vi "File.Move with Overwrite.vi"(8 "error in (no error)":errorcluster, 10 "Destination":path, 11 "Source":path) -> (0 "error out":errorcluster, 2 "Files Moved":i32, 3 "Destination Dup":path)   [LabVIEW 2024, in "EQMF.lvlib" / "File Utils.lvlib"]
uses:
  File Utils.lvlib
panel:
  out "Cmd":string
  out "RtnCode":i32
  out "StdErr":string
  out "StdOut":string
  # "If Source is Dir then Dest must be Dir\nFiles and subfolders are moved from the source path to the destination path.\nNOTE: In order to move a folder from a source location to a destination location, the source and destination path must include the folder."
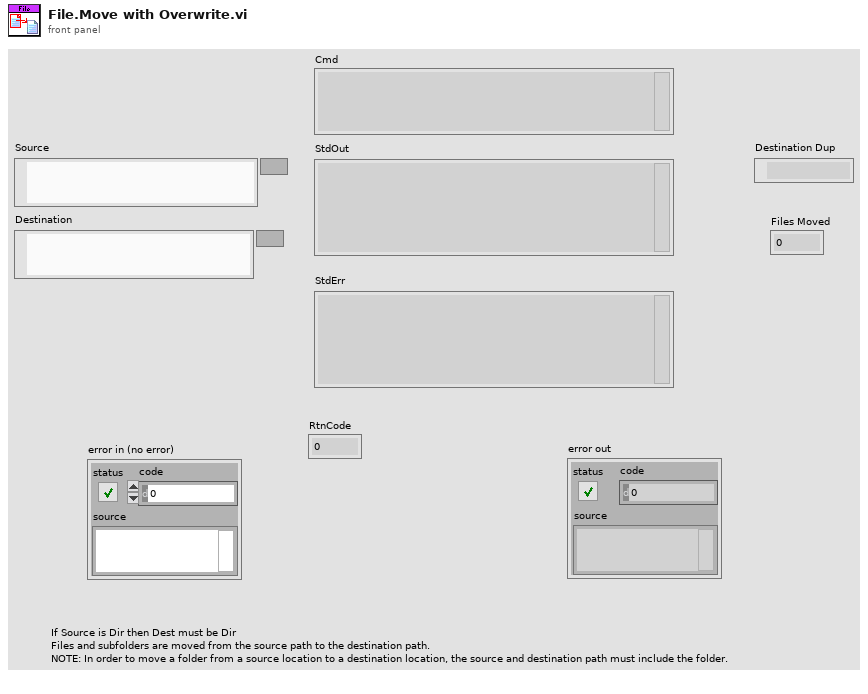
[diagram p1: front panel]
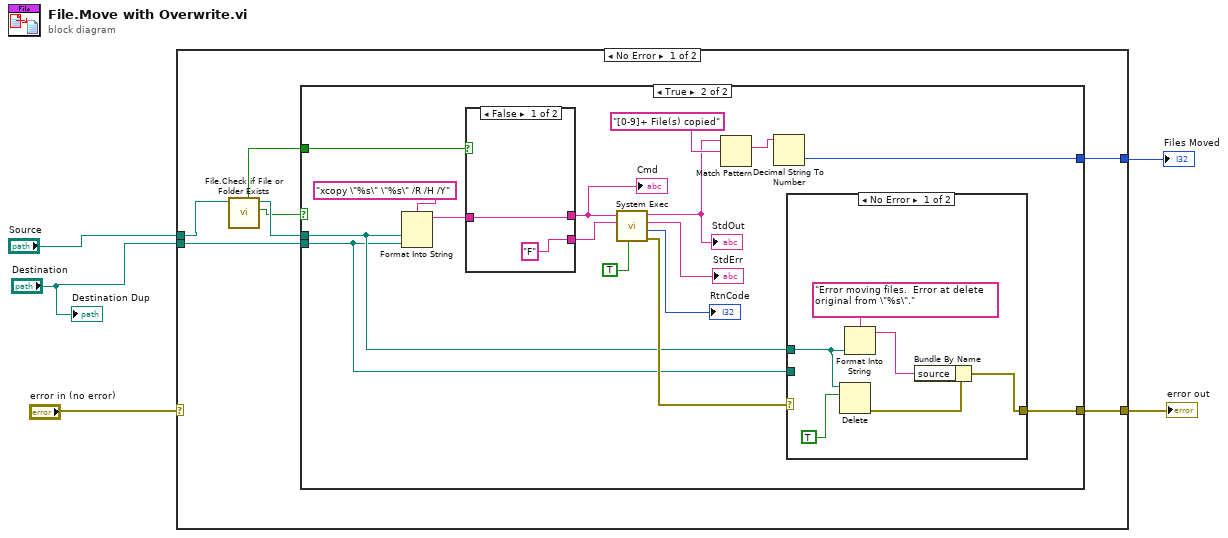
[diagram p0: block diagram]
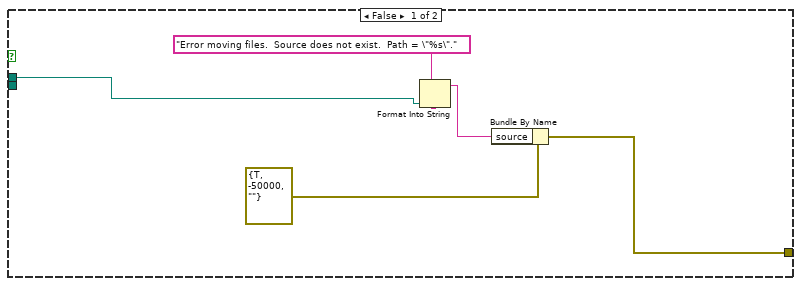
[diagram p2: hidden frame]
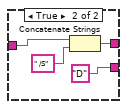
[diagram p3: hidden frame]
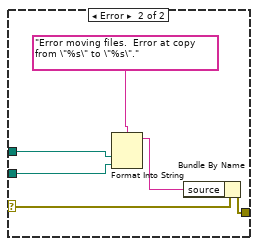
[diagram p4: hidden frame]
diagram:
  n1 = case shown="No Error" "error in (no error)" {
    selector: "error in (no error)" -> [_ w52]
    tunnel: "Source" -> [w9 _]
    tunnel: [w11 w52] -> w4
    tunnel: "Destination" -> [w10 _]
    tunnel: [w12 _] -> w1
    frame No Error {
      n2 = call "File.Check if File or Folder Exists.vi"("Path"=w9) -> ("Exists"=w7:bool, "Dup Path"=w8:path, "IsDir"=w6:bool)  [unwired: 6 in, 2 out]
      n3 = case shown="True" w7 {
        tunnel: [_ w27] -> w12
        tunnel: w8 -> [w14 w25]
        tunnel: [w13 w24] -> w11
        tunnel: w10 -> [_ w23]
        tunnel: w6 -> [_ w21]
        frame False {
          n4 = Format Into String(format string="Error moving files.  Source does not exist.  Path = \"%s\".", w14) -> (resulting string=w17:string)  [unwired: 2 in, 1 out]
          n5 = Bundle By Name(cluster=errorcluster {"status"=TRUE, "code"=-50000, "source"=""} ("error constant"), "source"=w17) -> (w13:errorcluster)
        }
        frame True {
          n6 = Format Into String(format string="xcopy \"%s\" \"%s\" /R /H /Y", w25, w23) -> (resulting string=w20:string)  [unwired: 2 in, 1 out]
          n7 = case shown="False" w21 {
            tunnel: w20 -> [w34 w37]
            tunnel: [w34 w39] -> w19
            tunnel: ["F" ("standard input") "D" ("standard input")] -> w18
            frame False {
            }
            frame True {
              n8 = Concatenate Strings(w37, " /S") -> (w39:string)
            }
          }
          "Cmd" <- w19
          n9 = call <vilib>:"System Exec.vi"("run minimized? (F)"=TRUE, "standard input"=w18, "command line"=w19) -> ("error out"=w26:errorcluster, "return code"=→"RtnCode":i32, "standard error"=→"StdErr":string, "standard output"=w29:string)  [unwired: 5 in]
          "StdOut" <- w29
          n10 = Match Pattern(string=w29, regular expression="[0-9]+ File(s) copied") -> (match substring=w28:string)  [unwired: 1 in, 3 out]
          n11 = Decimal String To Number(string=w28) -> (number=w27:i32)  [unwired: 2 in, 1 out]
          n12 = case shown="No Error" w26 {
            selector: w26 -> [_ w50]
            tunnel: w25 -> [w42 w48]
            tunnel: [w40 w51] -> w24
            tunnel: w23 -> [_ w47]
            frame No Error {
              n13 = Delete(path (use dialog)=w42, entire hierarchy (F)=TRUE) -> (error out=w41:errorcluster)  [unwired: 3 in, 2 out]
              n14 = Format Into String(format string="Error moving files.  Error at delete original from \"%s\".", w42) -> (resulting string=w44:string)  [unwired: 2 in, 1 out]
              n15 = Bundle By Name(cluster=w41, "source"=w44) -> (w40:errorcluster)
            }
            frame Error {
              n16 = Format Into String(format string="Error moving files.  Error at copy from \"%s\" to \"%s\".", w48, w47) -> (resulting string=w46:string)  [unwired: 2 in, 1 out]
              n17 = Bundle By Name(cluster=w50, "source"=w46) -> (w51:errorcluster)
            }
          }
        }
      }
    }
    frame Error {
    }
  }
  "error out" <- w4
  "Files Moved" <- w1
  "Destination Dup" <- "Destination"
